vi "S2DS_NewUpdatePlotData.vi"(3 "Present curve number XZ":i32, 4 "Plot data array":T1, 5 "Data":dbl[](array[numeric])) -> (1 "Plot data array out":T1)   [LabVIEW 2025]
uses:
  TYPE DEFS/S2DS_PlotCluster.ctl
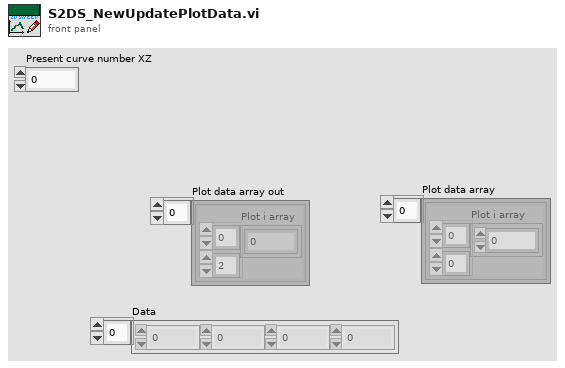
[diagram p1: front panel]
types:
  T1 = typedef "S2DS_PlotCluster.ctl" = cluster{"Plot i array":dbl[][]}[]
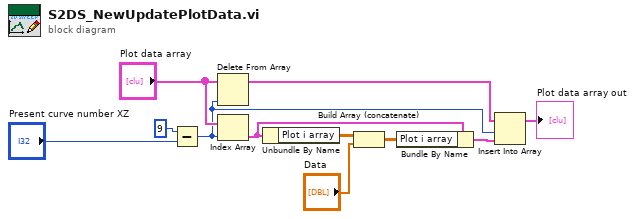
[diagram p0: block diagram]
diagram:
  n1 = Subtract(x=9, y="Present curve number XZ") -> (x-y=w1:i32)
  n2 = Delete From Array(array="Plot data array", index=w1) -> (array with subset deleted=w11:T1)  [unwired: 1 in, 1 out]
  n3 = Index Array(array="Plot data array", index=w1) -> (element=w5:cluster{"Plot i array":dbl[][]})
  n4 = Unbundle By Name(w5) -> ("Plot i array"=w10:dbl[][])
  n5 = Build Array (concatenate)(w10, "Data") -> (w4:dbl[][])
  n6 = Bundle By Name(cluster=w5, "Plot i array"=w4) -> (w3:cluster{"Plot i array":dbl[][]})
  n7 = Insert Into Array(array=w11, index=w1, new element=w3) -> (→"Plot data array out":T1)
